vi "On Stop.vi"(8 "error in (no error)":errorcluster, 10 "Data Queue":refnum<queue>, 11 "Settings in":T1) -> (0 "error out":errorcluster, 3 "Settings out":T1)   [LabVIEW 2021, in "Logging.lvlib"]
doc: "Empy the 'Data Queue' and write remaining data to disk, then close the log file."
uses:
  Logging.lvlib
  Settings/Settings.ctl
  Acquisition/Hardware Configuration.ctl
  Acquisition/Channel Settings.ctl
  Acquisition/IO Device.ctl
  Interval Timer/Repeat Interval.ctl
  Interval Timer/Interval Length.ctl
  Interval Timer/Interval Token.ctl
  Logging Configuration.ctl
  Diagnostics/Diagnostics Configuration.ctl
  controls/Acquired Data.ctl
  Acquisition/Acquisition.lvlib
  Interval Timer/Interval Timer.lvlib
  Diagnostics/Diagnostics.lvlib
  Settings/Settings.lvlib
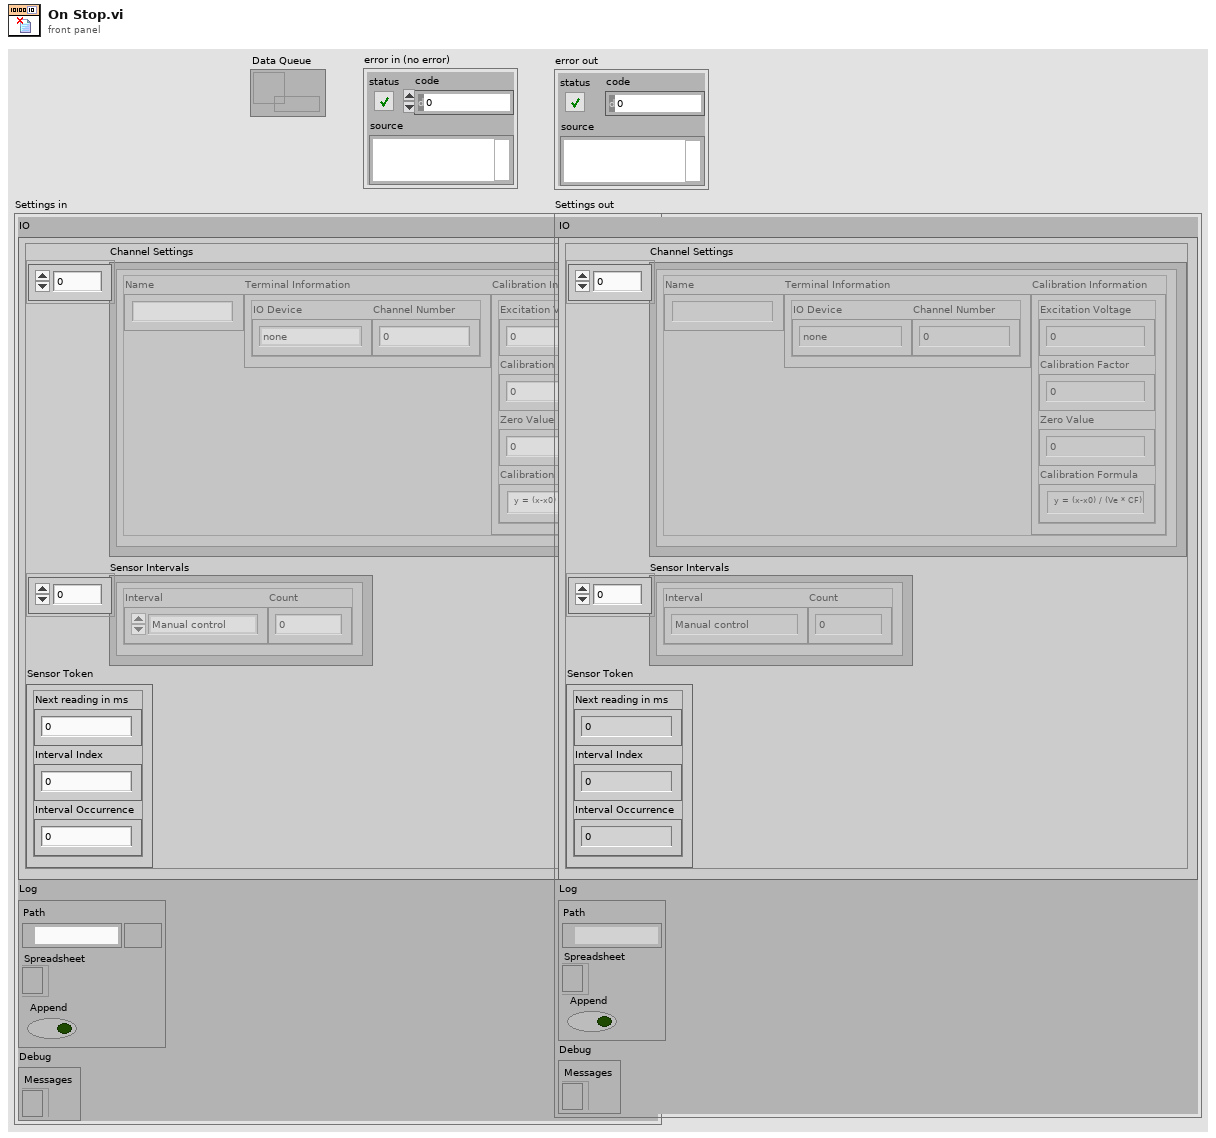
[diagram p1: front panel]
types:
  T1 = typedef "Settings.lvlib/Settings.ctl" = cluster{"IO":T2, "Log":T8, "Debug":T9}
  T2 = typedef "Acquisition.lvlib/Hardware Configuration.ctl" = cluster{"Channel Settings":T3[], "Sensor Intervals":T5[], "Sensor Token":T7}
  T3 = typedef "Acquisition.lvlib/Channel Settings.ctl" = cluster{"Name":string, "Terminal Information":cluster{"IO Device":T4, "Channel Number":i32}, "Calibration Information":cluster{"Excitation Voltage":dbl, "Calibration Factor":dbl, "Zero Value":dbl, "Calibration Formula":string}}
  T4 = typedef "Acquisition.lvlib/IO Device.ctl" = enum16{"none", "9219", "9401"}
  T5 = typedef "Interval Timer.lvlib/Repeat Interval.ctl" = cluster{"Interval":T6, "Count":i32}
  T6 = typedef "Interval Timer.lvlib/Interval Length.ctl" = enum16{"Manual control", "1 second", "10 seconds", "30 seconds", "60 seconds", "600 seconds", "1200 seconds", "3600 seconds"}
  T7 = typedef "Interval Timer.lvlib/Interval Token.ctl" = cluster{"Next reading in ms":u32, "Interval Index":i32, "Interval Occurrence":i32}
  T8 = typedef "Logging.lvlib/Logging Configuration.ctl" = cluster{"Path":path, "Spreadsheet":refnum<file>, "Append":bool}
  T9 = typedef "Diagnostics.lvlib/Diagnostics Configuration.ctl" = cluster{"Messages":refnum<file>}
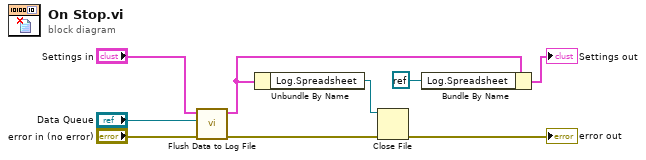
[diagram p0: block diagram]
diagram:
  n1 = call "Flush Data to Log File.vi"("error in (no error)"="error in (no error)", "Data Queue"="Data Queue", "Settings in"="Settings in") -> ("error out"=w3:errorcluster, "Settings out"=w1:T1)  [unwired: 7 in]
  n2 = Unbundle By Name(w1) -> ("Log.Spreadsheet"=w5:refnum<file>)
  n3 = Close File(refnum=w5, error in=w3) -> (error out=→"error out":errorcluster)  [unwired: 1 out]
  n4 = Bundle By Name(cluster=w1, "Log.Spreadsheet"=refnum<k0> refnum) -> (→"Settings out":T1)
